vi "Configure String Combo Box.vi"(7 "Operation Ctrl Ref":refnum<vi>, 8 "error in (no error)":errorcluster, 11 "Test in":refnum<class "Test.lvclass">) -> (0 "error out":errorcluster, 2 "Default test":string, 3 "Test out":refnum<class "Test.lvclass">)   [LabVIEW 2018, in "Test.lvclass"]
doc: "Configures the string combo box for Operation, using the correct display string and class name to build a new test"
uses:
  Test.lvclass
  Numeric Operations.ctl
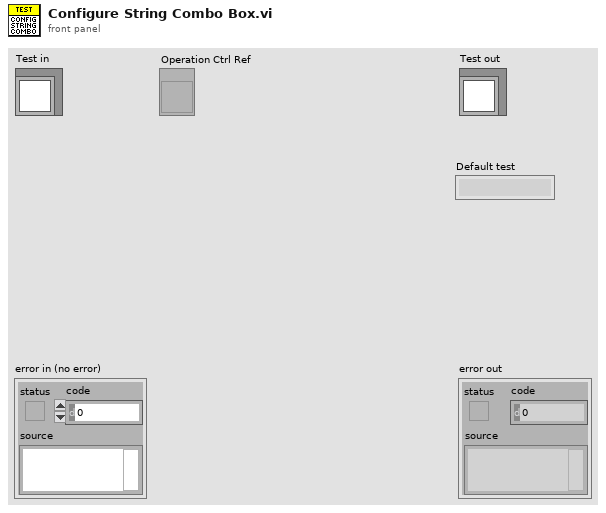
[diagram p1: front panel]
types:
  T1 = cluster{"Display String":string, "class name":string}
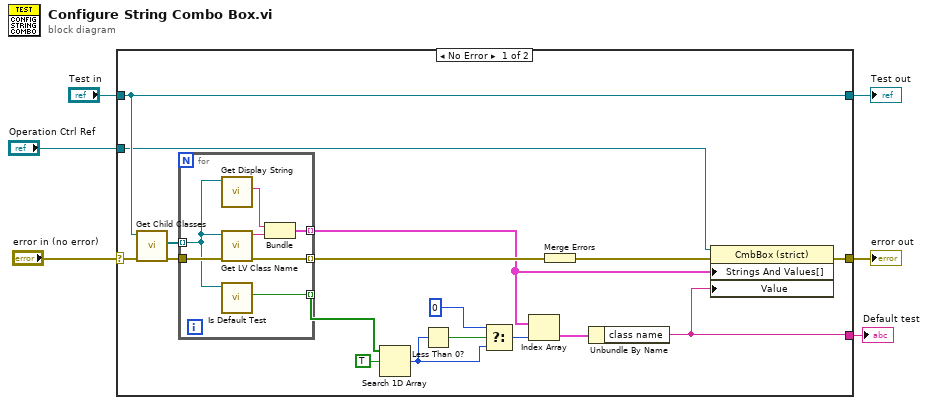
[diagram p0: block diagram]
diagram:
  n1 = case shown="No Error" "error in (no error)" {
    selector: "error in (no error)" -> [w23 w32]
    tunnel: [w20 w32] -> w5
    tunnel: [w22 w31] -> w3
    tunnel: "Test in" -> [w22 w31]
    tunnel: "Operation Ctrl Ref" -> [w16 _]
    tunnel: [w7 _] -> w1
    frame No Error {
      n2 = call "Get Child Classes.vi"("error in (no error)"=w23, "Test in"=w22) -> ("error out"=w19:errorcluster, "Child Classes"=w21:refnum<class "Test.lvclass">[])  [unwired: 8 in]
      n3 = for {
        tunnel: w21 -> [w25] mode=indexing
        tunnel: [w28] -> w13 mode=indexing
        tunnel: w19 -> [w27]
        tunnel: [w26] -> w18 mode=indexing
        tunnel: [w24] -> w15 mode=indexing
        n4 = call-dynamic "Get Display String.vi"("Test in"=w25) -> ("Display String"=w30:string)  [unwired: 10 in]
        n5 = call <vilib>:"Get LV Class Name.vi"("error in (no error)"=w27, "object"=w25) -> ("error out"=w26:errorcluster, "class name"=w29:string)  [unwired: 8 in]
        n6 = call-dynamic "Is Default Test.vi"("Test in"=w25) -> ("Is Default Test?"=w24:bool)  [unwired: 10 in]
        n7 = Bundle("Display String"=w30, "class name"=w29) -> (w28:T1)  [unwired: 1 in]
      }
      n8 = Search 1D Array(1D array=w15, element=TRUE) -> (index of element=w10:i32)  [unwired: 1 in]
      n9 = Less Than 0?(x=w10) -> (x < 0?=w11:bool)
      n10 = Select(t=0, s=w11, f=w10) -> (s? t:f=w8:i32)
      n11 = Index Array(array=w13, index=w8) -> (element=w12:T1)
      n12 = Merge Errors(w18) -> (w17:errorcluster)
      n13 = Unbundle By Name(w12) -> ("class name"=w7:string)
      n14 = property class="CmbBox (strict)"(reference=w16, error in=w17, "Strings And Values[]"=w13, "Value"=w7) -> (error out=w20:errorcluster)  [unwired: 1 out]
    }
    frame Error {
    }
  }
  "error out" <- w5
  "Test out" <- w3
  "Default test" <- w1
